vi "filter_result_yolov8.vi"(7 "confThreshold":sgl=0.5, 11 "2d_data":sgl[][](array[numeric])) -> (1 "index":i32[](array[numeric]), 2 "scores":sgl[](array[numeric]), 3 "filtered_data":sgl[][](array[numeric]))   [LabVIEW 2023]
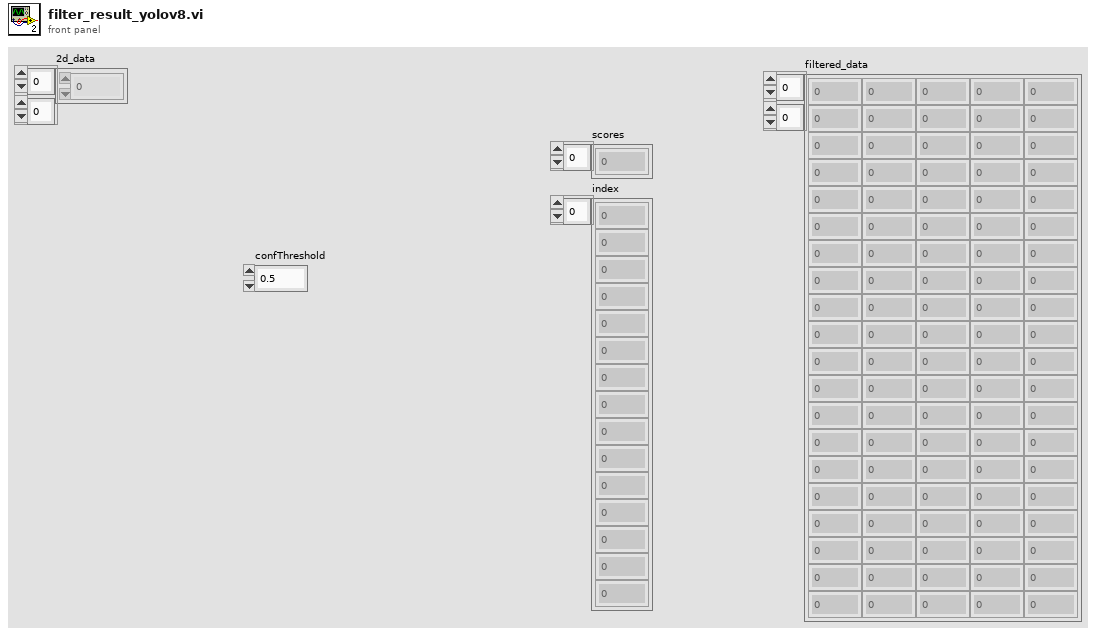
[diagram p1: front panel]
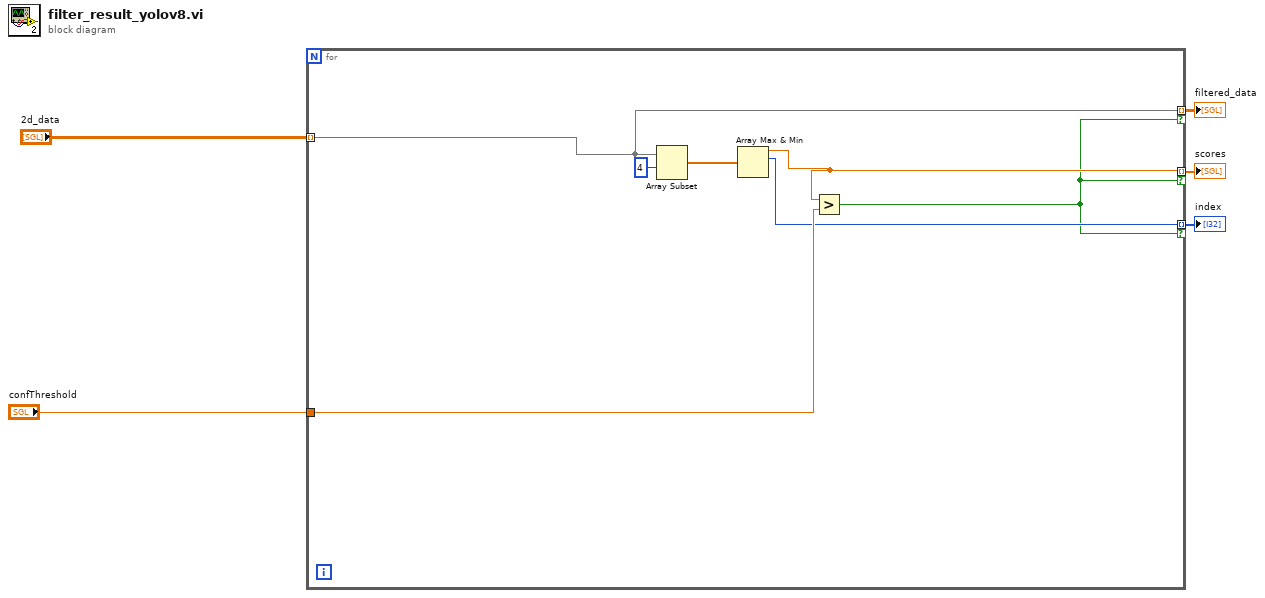
[diagram p0: block diagram]
diagram:
  n1 = for {
    tunnel: "2d_data" -> [w6] mode=indexing
    tunnel: "confThreshold" -> [w12]
    tunnel: [w6] -> w4 mode=indexing if=w9
    tunnel: [w11] -> w3 mode=indexing if=w9
    tunnel: [w10] -> w2 mode=indexing if=w9
    n2 = Array Subset(array=w6, index=4) -> (w7:sgl[])  [unwired: 1 in]
    n3 = Array Max & Min(array=w7) -> (max value=w11:sgl, max index (indices)=w10:i32)  [unwired: 2 out]
    n4 = Greater?(x=w11, y=w12) -> (0:w9:bool)
  }
  "filtered_data" <- w4
  "scores" <- w3
  "index" <- w2
